vi "Main.vi"() -> ()   [LabVIEW 2017]
uses:
  Controles/Estados.ctl
  Controles/Tipos de dato.ctl
  Controles/Inventario.ctl
  Controles/Producto.ctl
panel:
  in  "Ring":u16(ring)
  out "Restante":dbl
  in  "Productos":T1
  out "Cambio":dbl format="$ %.1f"
  in  "Stop":bool
  in  "Devuelve Dinero":bool
  out "Credito":dbl format="$ %.1f"
  in  "Monedas":T2
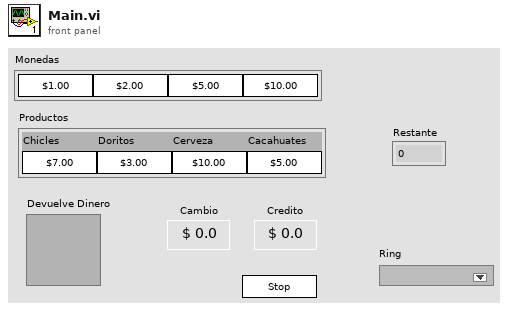
[diagram p1: front panel]
types:
  T1 = typedef "Producto.ctl" = cluster{"Chicles":bool, "Doritos":bool, "Cerveza":bool, "Cacahuates":bool}
  T2 = cluster{"1 Peso":bool, "2 Pesos":bool, "5 Pesos":bool, "10 Pesos":bool}
  T3 = typedef "Tipos de dato.ctl" = cluster{"Monedas":cluster{"1 Peso":bool, "2 Pesos":bool, "5 Pesos":bool, "10 Pesos":bool}, "Productos":T1, "Credito":dbl, "Devuelve Dinero":bool, "Stop":bool, "Cambio":dbl, "Costo del Producto":dbl, "Inventario":T4}
  T4 = typedef "Inventario.ctl" = cluster{"Chicles":dbl, "Doritos":dbl, "Cerveza":dbl, "Cacahuates":dbl}
  T5 = typedef "Estados.ctl" = enum16{"Esperar moneda", "Incrementar Credito", "Seleccionar Productos", "Credito Vs Costo", "Regresar Dinero/Cambio", "Entregar producto", "Revisa/Actualiza Inventario"}
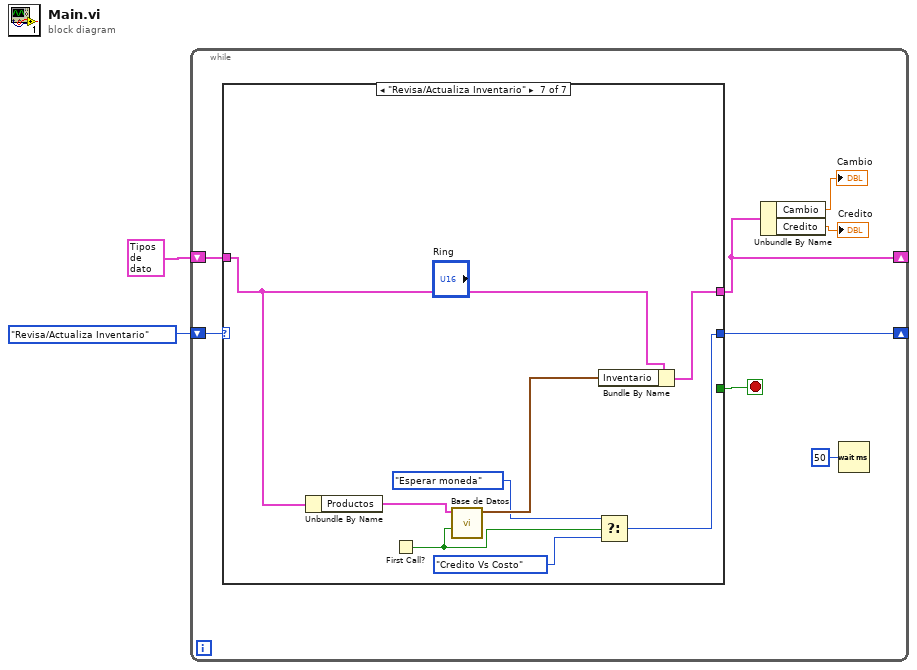
[diagram p0: block diagram]
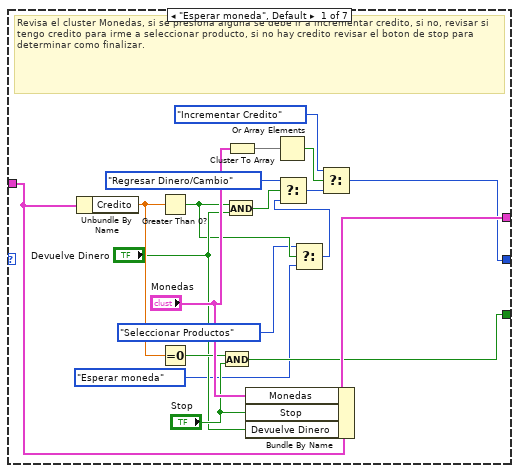
[diagram p2: hidden frame]
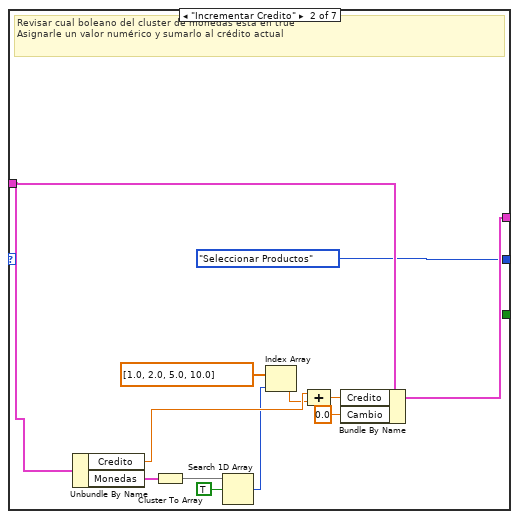
[diagram p3: hidden frame]
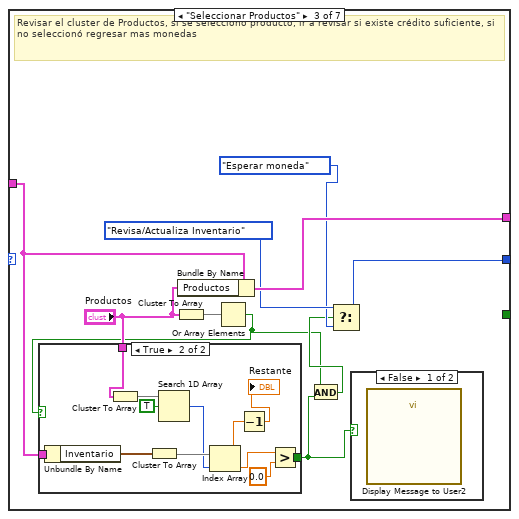
[diagram p4: hidden frame]
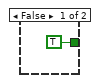
[diagram p5: hidden frame]
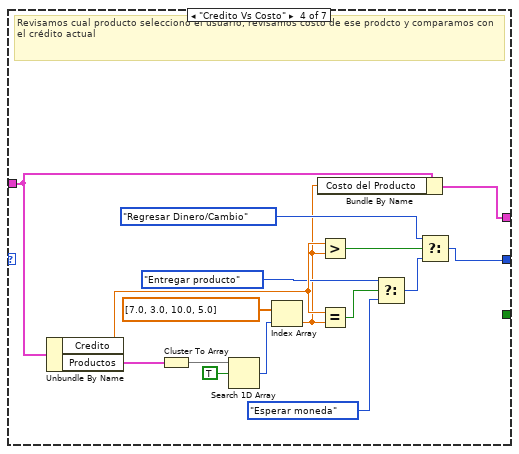
[diagram p7: hidden frame]
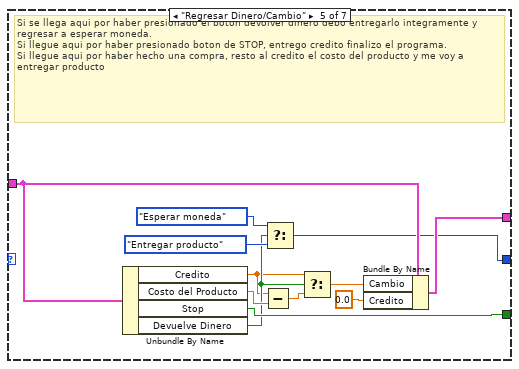
[diagram p8: hidden frame]
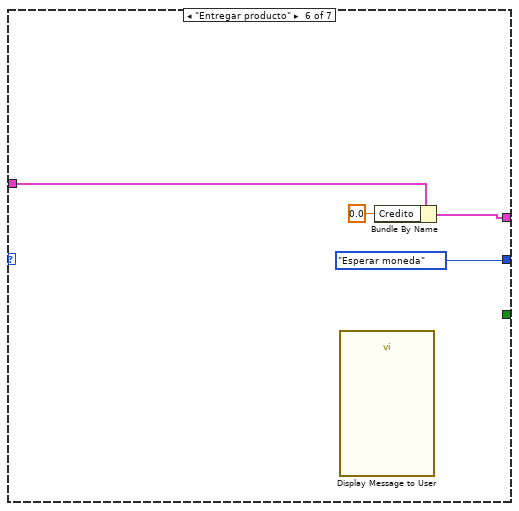
[diagram p9: hidden frame]
diagram:
  n1 = while {
    shift-right: [w6] -> _
    shift-left: Estados."Revisa/Actualiza Inventario" -> [w10]
    shift-right: [w8] -> _
    shift-left: T3 {"Monedas"={"1 Peso"=FALSE, "2 Pesos"=FALSE, "5 Pesos"=FALSE, "10 Pesos"=FALSE}, "Productos"={"Chicles"=FALSE, "Doritos"=FALSE, "Cerveza"=FALSE, "Cacahuates"=FALSE}, "Credito"=0.0, "Devuelve Dinero"=FALSE, "Stop"=FALSE, "Cambio"=0.0, "Costo del Producto"=0.0, "Inventario"={"Chicles"=0.0, "Doritos"=0.0, "Cerveza"=0.0, "Cacahuates"=0.0}} ("Cluster") -> [w9]
    stop <- w5 stop-if-true
    n2 = case shown="\"Revisa/Actualiza Inventario\"" w10 {
      tunnel: w9 -> [w26 w34 w46 w66 w90 w93 w103]
      tunnel: [w27 w32 w51 w64 w88 w94 w102] -> w8
      tunnel: [w24 Estados."Seleccionar Productos" ("f") w47 w67 w84 Estados."Esperar moneda" w96] -> w6
      tunnel: [w21 _ _ _ w85 _ _] -> w5
      frame "Esperar moneda", Default {
        # "Revisa el cluster Monedas, si se presiona alguna se debe ir a incrementar credito, si no, revisar si tengo credito para irme a seleccionar producto, si no hay credito revisar el boton de stop para determinar como finalizar."
        n3 = Unbundle By Name(w26) -> ("Credito"=w19:dbl)
        n4 = Greater Than 0?(x=w19) -> (x > 0?=w14:bool)
        n5 = Equal To 0?(x=w19) -> (x = 0?=w22:bool)
        n6 = And(x=w22, y="Stop") -> (x .and. y?=w21:bool)
        n7 = And(x=w14, y="Devuelve Dinero") -> (x .and. y?=w16:bool)
        n8 = Cluster To Array(cluster="Monedas") -> (array=w29:bool[])
        n9 = Bundle By Name(cluster=w26, "Monedas"="Monedas", "Stop"="Stop", "Devuelve Dinero"="Devuelve Dinero") -> (w27:T3)
        n10 = Or Array Elements(Boolean array=w29) -> (logical OR=w23:bool)
        n11 = Select(t=Estados."Seleccionar Productos" ("f"), s=w14, f=Estados."Esperar moneda") -> (s? t:f=w11:T5)
        n12 = Select(t=Estados."Regresar Dinero/Cambio", s=w16, f=w11) -> (s? t:f=w18:T5)
        n13 = Select(t=Estados."Incrementar Credito", s=w23, f=w18) -> (s? t:f=w24:T5)
      }
      frame "Incrementar Credito" {
        # "Revisar cual boleano del cluster de monedas está en true\nAsignarle un valor numérico y sumarlo al crédito actual"
        n14 = Unbundle By Name(w34) -> ("Credito"=w38:dbl, "Monedas"=w41:T2)
        n15 = Cluster To Array(cluster=w41) -> (array=w40:bool[])
        n16 = Search 1D Array(1D array=w40, element=TRUE) -> (index of element=w37:i32)  [unwired: 1 in]
        n17 = Index Array(array=dbl[] [1.0, 2.0, 5.0, 10.0], index=w37) -> (element=w35:dbl)
        n18 = Compound Arithmetic op=ADD(w38, w35) -> (w33:dbl)
        n19 = Bundle By Name(cluster=w34, "Credito"=w33, "Cambio"=0.0) -> (w32:T3)
      }
      frame "Seleccionar Productos" {
        # "Revisar el cluster de Productos, si se seleccionó producto, ir a revisar si existe crédito suficiente, si no seleccionó regresar mas monedas"
        n20 = Cluster To Array(cluster="Productos") -> (array=w50:bool[])
        n21 = Bundle By Name(cluster=w46, "Productos"="Productos") -> (w51:T3)
        n22 = Or Array Elements(Boolean array=w50) -> (logical OR=w42:bool)
        n23 = case shown="True" w42 {
          tunnel: w46 -> [_ w63]
          tunnel: "Productos" -> [_ w58]
          tunnel: [TRUE w54] -> w43
          frame False {
          }
          frame True {
            n24 = Unbundle By Name(w63) -> ("Inventario"=w62:T4)
            n25 = Cluster To Array(cluster=w58) -> (array=w59:bool[])
            n26 = Cluster To Array(cluster=w62) -> (array=w61:dbl[])
            n27 = Search 1D Array(1D array=w59, element=TRUE) -> (index of element=w60:i32)  [unwired: 1 in]
            n28 = Index Array(array=w61, index=w60) -> (element=w56:dbl)
            n29 = Decrement(x=w56) -> (x-1=→"Restante":dbl)
            n30 = Greater?(x=w56, y=0.0) -> (0:w54:bool)
          }
        }
        n31 = And(x=w42, y=w43) -> (x .and. y?=w44:bool)
        n32 = Select(t=Estados."Revisa/Actualiza Inventario", s=w44, f=Estados."Esperar moneda") -> (s? t:f=w47:T5)
        n33 = case shown="False" w43 {
          frame False {
            n34 = call "Display Message to User2"() -> ()  [unwired: 10 in, 2 out]
          }
          frame True {
          }
        }
      }
      frame "Credito Vs Costo" {
        # "Revisamos cual producto seleccionó el usuario, revisamos costo de ese prodcto y comparamos con el crédito actual"
        n35 = Unbundle By Name(w66) -> ("Credito"=w72:dbl, "Productos"=w79:T1)
        n36 = Cluster To Array(cluster=w79) -> (array=w78:bool[])
        n37 = Search 1D Array(1D array=w78, element=TRUE) -> (index of element=w76:i32)  [unwired: 1 in]
        n38 = Index Array(array=dbl[] [7.0, 3.0, 10.0, 5.0], index=w76) -> (element=w65:dbl)
        n39 = Bundle By Name(cluster=w66, "Costo del Producto"=w65) -> (w64:T3)
        n40 = Greater?(x=w72, y=w65) -> (0:w74:bool)
        n41 = Equal?(x=w72, y=w65) -> (x = y?=w71:bool)
        n42 = Select(t=Estados."Entregar producto", s=w71, f=Estados."Esperar moneda") -> (s? t:f=w68:T5)
        n43 = Select(t=Estados."Regresar Dinero/Cambio", s=w74, f=w68) -> (s? t:f=w67:T5)
      }
      frame "Regresar Dinero/Cambio" {
        # "Si se llega aqui por haber presionado el boton devolver dinero debo entregarlo integramente y regresar a esperar moneda.\nSi llegue aqui por haber presionado boton de STOP, entrego credito finalizo el programa.\nSi llegue aqui por haber hecho una compra, resto al credito el costo del producto y me voy a entregar producto"
        n44 = Unbundle By Name(w90) -> ("Credito"=w80:dbl, "Costo del Producto"=w91:dbl, "Stop"=w85:bool, "Devuelve Dinero"=w83:bool)
        n45 = Subtract(x=w80, y=w91) -> (x-y=w82:dbl)
        n46 = Select(t=Estados."Esperar moneda", s=w83, f=Estados."Entregar producto") -> (s? t:f=w84:T5)
        n47 = Select(t=w80, s=w83, f=w82) -> (s? t:f=w81:dbl)
        n48 = Bundle By Name(cluster=w90, "Cambio"=w81, "Credito"=0.0) -> (w88:T3)
      }
      frame "Entregar producto" {
        n49 = call "Display Message to User"() -> ()  [unwired: 10 in, 2 out]
        n50 = Bundle By Name(cluster=w93, "Credito"=0.0) -> (w94:T3)
      }
      frame "Revisa/Actualiza Inventario" {
        n51 = Unbundle By Name(w103) -> ("Productos"=w101:T1)
        n52 = First Call?() -> (First Call?: T/F=w99:bool)
        n53 = call "Base de Datos.vi"("Boolean"=w99, "Productos"=w101) -> ("Inventario"=w100:T4)  [unwired: 9 in]
        n54 = Bundle By Name(cluster=w103, "Inventario"=w100) -> (w102:T3)
        n55 = Select(t=Estados."Esperar moneda", s=w99, f=Estados."Credito Vs Costo") -> (s? t:f=w96:T5)
      }
    }
    n56 = Unbundle By Name(w8) -> ("Cambio"=→"Cambio":dbl, "Credito"=→"Credito":dbl)
    n57 = Wait (ms)(milliseconds to wait=u32 50) -> ()  [unwired: 1 out]
  }
